vi "SCrc_CalculateCRC8H2F (Hella).vi"(1 "DataIDList":u8[](array[numeric]), 2 "Counter":u8, 3 "Data":u8[](array[numeric]), 5 "SCrc_Length":u8, 7 "SCrc_StartValue8H2F IN":u8, 9 "SCrc_IsFirstCall":bool) -> (8 "SCrc_StartValue8H2F OUT":u8)   [LabVIEW 2013]
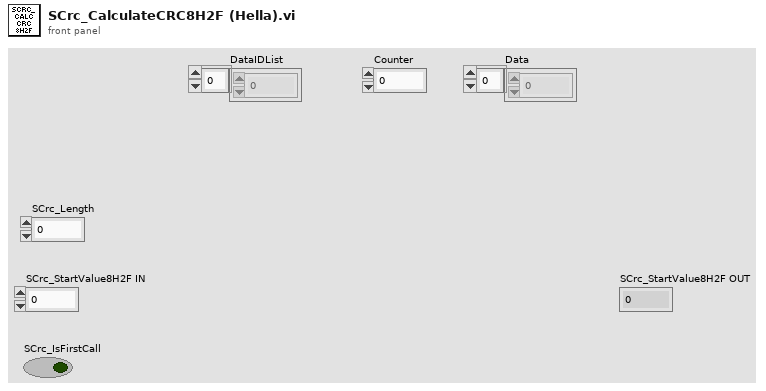
[diagram p1: front panel]
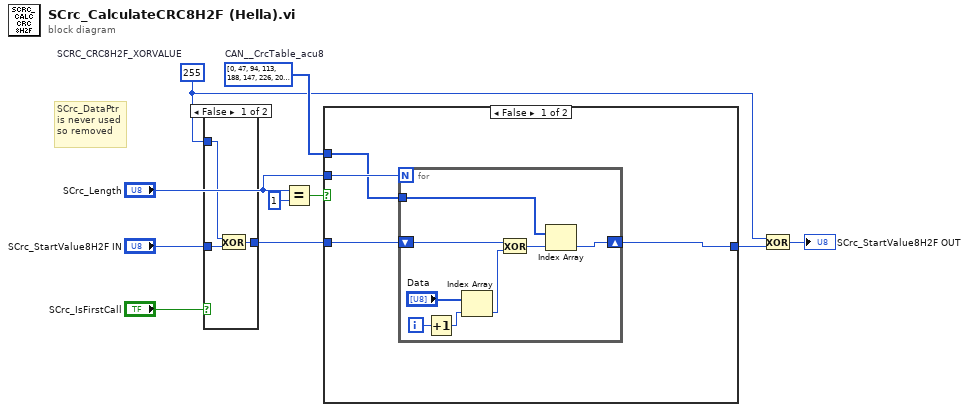
[diagram p0: block diagram]
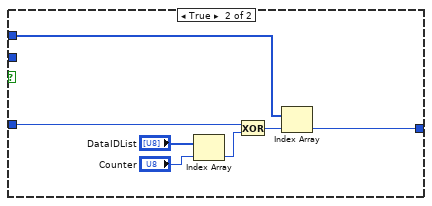
[diagram p2: hidden frame]
diagram:
  w4 = u8 255  # SCRC_CRC8H2F_XORVALUE
  w7 = u8[] [0, 47, 94, 113, 188, 147, 226, 205, 87, 120, 9, 38, 235, 196, 181, 154, 174, 129, 240, 223, 18, 61, 76, 99, 249, 214, 167, 136, 69, 106, 27, 52, 115, 92, 45, 2, 207, 224, 145, 190, 36, 11, 122, 85, 152, 183, 198, 233, 221, 242, 131, 172, 97, 78, 63, 16, 138, 165, 212, 251, 54, 25, 104, 71, 230, 201, 184, 151, 90, 117, 4, 43, 177, 158, 239, 192, 13, 34, 83, 124, 72, 103, 22, 57, 244, 219, 170, 133, 31, 48, 65, 110, 163, 140, 253, 210, 149, 186, 203, 228, 41, 6, 119, 88, 194, 237, 156, 179, 126, 81, 32, 15, 59, 20, 101, 74, 135, 168, 217, 246, 108, 67, 50, 29, 208, 255, 142, 161, 227, 204, 189, 146, 95, 112, 1, 46, 180, 155, 234, 197, 8, 39, 86, 121, 77, 98, 19, 60, 241, 222, 175, 128, 26, 53, 68, 107, 166, 137, 248, 215, 144, 191, 206, 225, 44, 3, 114, 93, 199, 232, 153, 182, 123, 84, 37, 10, 62, 17, 96, 79, 130, 173, 220, 243, 105, 70, 55, 24, 213, 250, 139, 164, 5, 42, 91, 116, 185, 150, 231, 200, 82, 125, 12, 35, 238, 193, 176, 159, 171, 132, 245, 218, 23, 56, 73, 102, 252, 211, 162, 141, 64, 111, 30, 49, 118, 89, 40, 7, 202, 229, 148, 187, 33, 14, 127, 80, 157, 178, 195, 236, 216, 247, 134, 169, 100, 75, 58, 21, 143, 160, 209, 254, 51, 28, 109, 66]  # CAN__CrcTable_acu8
  # "SCrc_DataPtr\nis never used\nso removed"
  n1 = case shown="False" "SCrc_IsFirstCall" {
    tunnel: "SCrc_StartValue8H2F IN" -> [w13 _]
    tunnel: w4 -> [w12 w14]
    tunnel: [w11 w14] -> w1
    frame False {
      n2 = Exclusive Or(1:w13, 2:w12) -> (0:w11:u8)
    }
    frame True {
    }
  }
  n3 = Equal?(x="SCrc_Length", y=u8 1) -> (x = y?=w2:bool)
  n4 = case shown="False" w2 {
    tunnel: w1 -> [w17 w28]
    tunnel: w7 -> [w16 w31]
    tunnel: [w15 w27] -> w6
    tunnel: "SCrc_Length" -> [w18 _]
    frame False {
      n5 = for {
        N: w18 -> [_]
        tunnel: w16 -> [w21]
        shift-right: [w19] -> w15
        shift-left: w17 -> [w23]
        i -> [w24]
        n6 = Increment(x=w24) -> (x+1=w25:i32)
        n7 = Index Array(array="Data", index=w25) -> (element=w22:u8)
        n8 = Exclusive Or(1:w22, 2:w23) -> (0:w20:u8)
        n9 = Index Array(array=w21, index=w20) -> (element=w19:u8)
      }
    }
    frame True {
      n10 = Index Array(array="DataIDList", index="Counter") -> (element=w29:u8)
      n11 = Exclusive Or(1:w29, 2:w28) -> (0:w30:u8)
      n12 = Index Array(array=w31, index=w30) -> (element=w27:u8)
    }
  }
  n13 = Exclusive Or(1:w6, 2:w4) -> (0:→"SCrc_StartValue8H2F OUT":u8)
